vi "Adjust Phase Scale.vi"(6 "Show Scale?":bool, 8 "error in (no error)":errorcluster, 9 "Plot Area Bounds":T3, 10 "Origin Coords":T4, 11 "Control Ref Cluster":T1) -> (0 "error out":errorcluster, 1 "Dup Plot Area Bounds":T3, 2 "Dup Origin Coords":T4, 3 "Dup Control Ref Cluster":T1)   [LabVIEW 2017, in "2D Compass.lvclass"]
uses:
  <vilib>/Math Plots/2D Math Plots/2D Compass/2D Compass/2D Compass.lvclass
  <vilib>/Utility/miscctls.llb/LVPoint32TypeDef.ctl
  <vilib>/Math Plots/2D Math Plots/2D Plot/Action String/2DMathPlot Ctrl Act Cluster.ctl
  <vilib>/Math Plots/2D Math Plots/2D Plot/Action String/2DMathPlot State Class.ctl
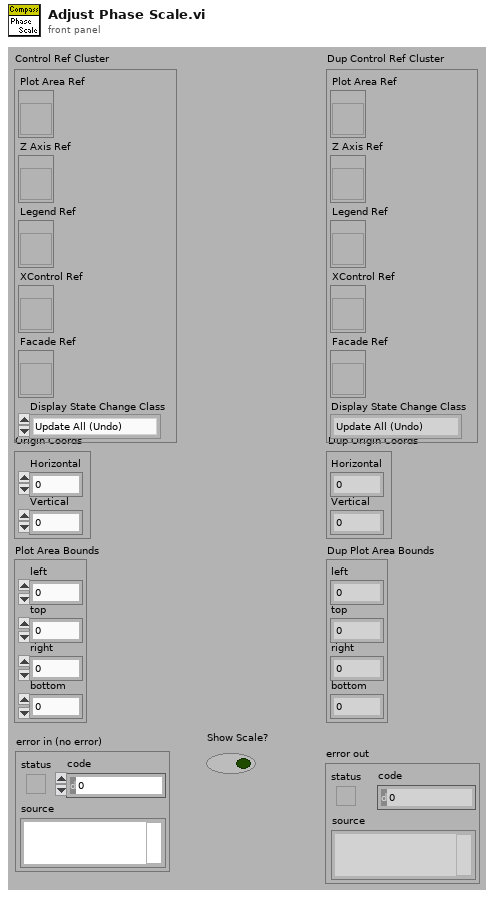
[diagram p1: front panel]
types:
  T1 = typedef "2DMathPlot Ctrl Act Cluster.ctl" = cluster{"Plot Area Ref":refnum<vi>, "Z Axis Ref":refnum<vi>, "Legend Ref":refnum<vi>, "XControl Ref":refnum<vi>, "Facade Ref":refnum<vi>, "Display State Change Class":T2}
  T2 = typedef "2DMathPlot State Class.ctl" = enum16{"Update All (Undo)", "Update General", "Update Appearance", "Update Format", "Update Scale", "Update Marker", "Update Cursor", "None"}
  T3 = cluster{"left":i32, "top":i32, "right":i32, "bottom":i32}
  T4 = typedef "LVPoint32TypeDef.ctl" = cluster{"Horizontal":i32, "Vertical":i32}
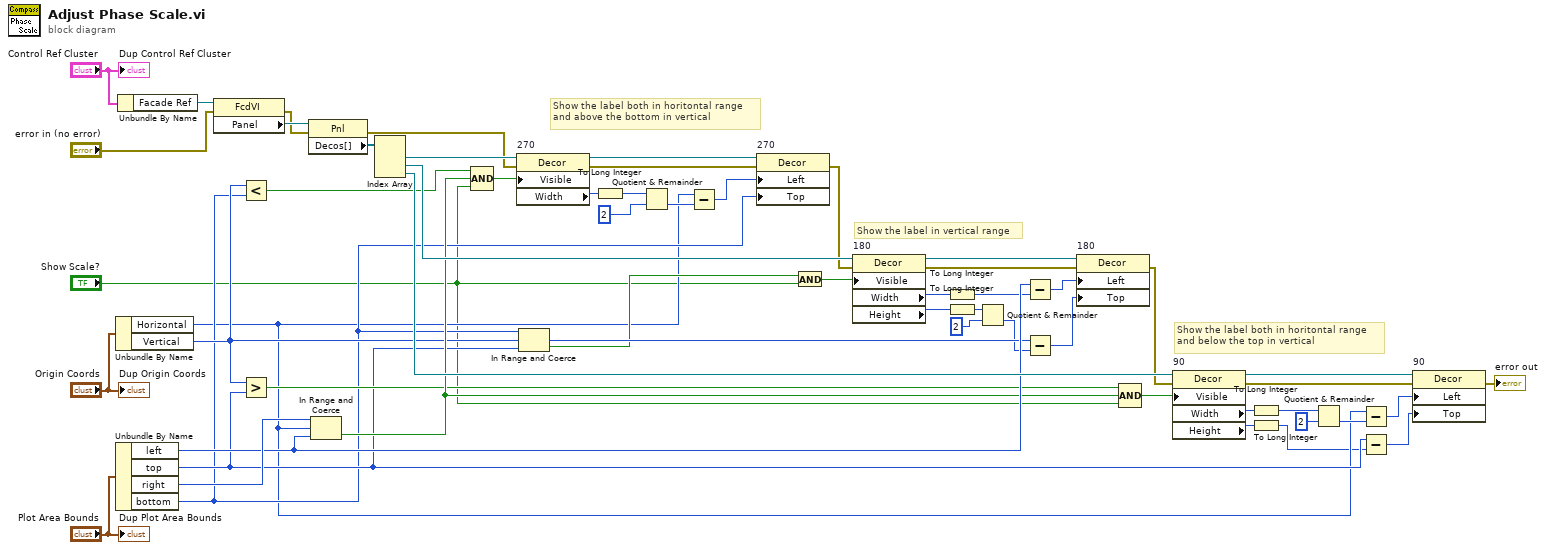
[diagram p0: block diagram]
diagram:
  # "Show the label both in horitontal range\nand below the top in vertical"
  # "Show the label both in horitontal range\nand above the bottom in vertical"
  # "Show the label in vertical range"
  n1 = Unbundle By Name("Origin Coords") -> ("Horizontal"=w8:i32, "Vertical"=w41:i32)
  n2 = Unbundle By Name("Plot Area Bounds") -> ("left"=w47:i32, "top"=w40:i32, "right"=w48:i32, "bottom"=w29:i32)
  n3 = Unbundle By Name("Control Ref Cluster") -> ("Facade Ref"=w1:refnum<vi>)
  n4 = property class="FcdVI"(reference=w1, error in="error in (no error)") -> (error out=w54:errorcluster, "Panel"=w56:refnum<vi>)  [unwired: 1 out]
  n5 = Less?(x=w41, y=w29) -> (x < y?=w43:bool)
  n6 = Greater?(x=w41, y=w40) -> (0:w42:bool)
  n7 = property class="Pnl"(reference=w56, error in=w54) -> (error out=w37:errorcluster, "Decos[]"=w55:refnum<vi>[])  [unwired: 1 out]
  n8 = In Range and Coerce(upper limit=w48, x=w8, lower limit=w47) -> (In Range?=w45:bool)  [unwired: 1 out]
  n9 = Index Array(array=w55) -> (element #1=w49:refnum<vi>, element #2=w50:refnum<vi>, element #3=w51:refnum<vi>)  [unwired: 3 in]
  n10 = Compound Arithmetic op=AND(w43, w45, "Show Scale?") -> (w46:bool)
  n11 = property on="270" class="Decor"(reference=w49, error in=w37, "Visible"=w46) -> (reference out=w34:refnum<vi>, error out=w36:errorcluster, "Width"=w32:u32)
  n12 = In Range and Coerce(upper limit=w29, x=w41, lower limit=w40) -> (In Range?=w39:bool)  [unwired: 1 out]
  n13 = To Long Integer(number=w32) -> (32bit integer=w30:i32)
  n14 = Quotient & Remainder(x=w30, y=2) -> (floor(x/y)=w31:i32)  [unwired: 1 out]
  n15 = Subtract(x=w8, y=w31) -> (x-y=w28:i32)
  n16 = property on="270" class="Decor"(reference=w34, error in=w36, "Left"=w28, "Top"=w29) -> (error out=w35:errorcluster)  [unwired: 1 out]
  n17 = And(x=w39, y="Show Scale?") -> (x .and. y?=w4:bool)
  n18 = property on="180" class="Decor"(reference=w50, error in=w35, "Visible"=w4) -> (reference out=w27:refnum<vi>, error out=w26:errorcluster, "Width"=w24:u32, "Height"=w21:u32)
  n19 = To Long Integer(number=w24) -> (32bit integer=w22:i32)
  n20 = To Long Integer(number=w21) -> (32bit integer=w20:i32)
  n21 = Quotient & Remainder(x=w20, y=2) -> (floor(x/y)=w18:i32)  [unwired: 1 out]
  n22 = Subtract(x=w47, y=w22) -> (x-y=w23:i32)
  n23 = Subtract(x=w41, y=w18) -> (x-y=w17:i32)
  n24 = property on="180" class="Decor"(reference=w27, error in=w26, "Left"=w23, "Top"=w17) -> (error out=w25:errorcluster)  [unwired: 1 out]
  n25 = Compound Arithmetic op=AND(w42, w45, "Show Scale?") -> (w44:bool)
  n26 = property on="90" class="Decor"(reference=w51, error in=w25, "Visible"=w44) -> (reference out=w15:refnum<vi>, error out=w16:errorcluster, "Width"=w11:u32, "Height"=w7:u32)
  n27 = To Long Integer(number=w11) -> (32bit integer=w13:i32)
  n28 = To Long Integer(number=w7) -> (32bit integer=w5:i32)
  n29 = Quotient & Remainder(x=w13, y=2) -> (floor(x/y)=w10:i32)  [unwired: 1 out]
  n30 = Subtract(x=w8, y=w10) -> (x-y=w9:i32)
  n31 = Subtract(x=w40, y=w5) -> (x-y=w6:i32)
  n32 = property on="90" class="Decor"(reference=w15, error in=w16, "Left"=w9, "Top"=w6) -> (error out=→"error out":errorcluster)  [unwired: 1 out]
  "Dup Origin Coords" <- "Origin Coords"
  "Dup Plot Area Bounds" <- "Plot Area Bounds"
  "Dup Control Ref Cluster" <- "Control Ref Cluster"
